vi "Convert to Waveforms (Multiple Lines).vi"(0 "data in":sgl[][](array[numeric]) format="%#.21g", 2 "reset? (F)":bool, 5 "sample rate [Hz]":sgl=9600.0 format="%#.6g", 7 "timestamp":timestamp, 9 "system info in":refnum<class "EP System Info.lvclass">, 11 "error in (no error)":errorcluster) -> (4 "voltage waveforms":waveform(dbl)[](array[waveform]), 6 "current waveforms":waveform(dbl)[](array[waveform]), 10 "system info out":refnum<class "EP System Info.lvclass">, 14 "interval length [s]":dbl, 15 "error out":errorcluster)   [LabVIEW 2014, in "NI_EP_Power Quality.lvlib"]
doc: "Converts resampled voltage and current data to voltage and current waveforms of different line configurations. This VI also arranges the order of the elements in the waveforms of each three-phase electrical power system for further measurement. For example, the orders are A-B-C-N for the four-channel method and A-B-C for the three-channel method. You must manually select the polymorphic instance you want to use."
uses:
  <vilib>/addons/Electrical Power/PQ/NI_EP_Power Quality.lvlib
  <vilib>/addons/Electrical Power/PQ/Common/Classes/System Info/EP System Info.lvclass
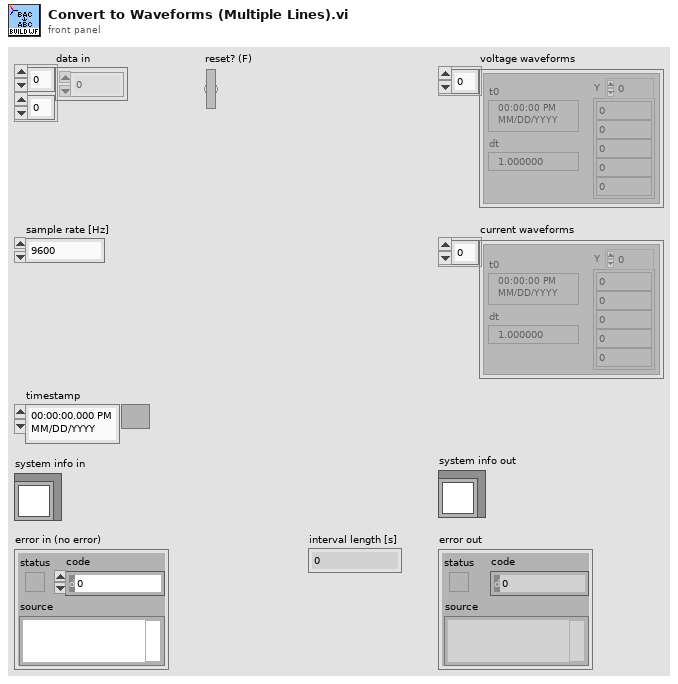
[diagram p1: front panel]
types:
  T1 = typedef "NI_EP_Power Quality.lvlib/ep_Channels Config.ctl" = cluster{"3-phase system ID":string, "physical channels":cluster{"channel phase":T2, "physical channel index":u16}[]}
  T2 = typedef "NI_EP_Power Quality.lvlib/ep_Channel Phase.ctl" = u16
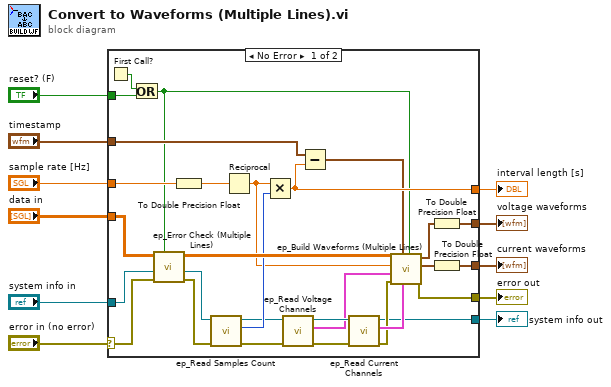
[diagram p0: block diagram]
diagram:
  n1 = case shown="No Error" "error in (no error)" {
    selector: "error in (no error)" -> [w32 w42]
    tunnel: "sample rate [Hz]" -> [w40 _]
    tunnel: "timestamp" -> [w39 _]
    tunnel: [w38 _] -> w9
    tunnel: [w24 _] -> w8
    tunnel: [w23 _] -> w7
    tunnel: "data in" -> [w31 _]
    tunnel: [w35 w42] -> w5
    tunnel: [w16 w41] -> w4
    tunnel: "reset? (F)" -> [w28 _]
    tunnel: "system info in" -> [w29 w41]
    frame No Error {
      n2 = First Call?() -> (First Call?: T/F=w33:bool)
      n3 = Or(x=w33, y=w28) -> (x .or. y?=w12:bool)
      n4 = call <vilib>:"ep_Error Check (Multiple Lines).vi"("reset? (F)"=w12, "error in (no error)"=w32, "system info in"=w29, "data in"=w31) -> ("error out"=w26:errorcluster, "system info out"=w27:refnum<class "EP System Info.lvclass">, "data out"=w30:sgl[][])  [unwired: 5 in]
      n5 = To Double Precision Float(number=w40) -> (double precision float=w34:dbl)
      n6 = call <vilib>:"ep_Read Samples Count.vi"("error in (no error)"=w26, "system info in"=w27) -> ("error out"=w20:errorcluster, "basic calc. interval (samples)"=w25:i32, "system info out"=w22:refnum<class "EP System Info.lvclass">)  [unwired: 5 in, 2 out]
      n7 = Reciprocal(x=w34) -> (1/x=w15:dbl)
      n8 = Multiply(x=w15, y=w25) -> (x*y=w38:dbl)
      n9 = call <vilib>:"ep_Read Voltage Channels.vi"("error in (no error)"=w20, "system info in"=w22) -> ("error out"=w19:errorcluster, "voltage channels"=w13:T1[], "system info out"=w21:refnum<class "EP System Info.lvclass">)  [unwired: 7 in]
      n10 = Subtract(x=w39, y=w38) -> (x-y=w14:timestamp)
      n11 = call <vilib>:"ep_Read Current Channels.vi"("error in (no error)"=w19, "system info in"=w21) -> ("error out"=w17:errorcluster, "current channels"=w18:T1[], "system info out"=w16:refnum<class "EP System Info.lvclass">)  [unwired: 7 in]
      n12 = call <vilib>:"ep_Build Waveforms (Multiple Lines).vi"("reset? (F)"=w12, "current channels"=w18, "t0"=w14, "error in (no error)"=w17, "voltage channels"=w13, "dt"=w15, "AI data"=w30) -> ("error out"=w35:errorcluster, "current waveforms"=w36:waveform(sgl)[], "voltage waveforms"=w37:waveform(sgl)[])  [unwired: 2 in]
      n13 = To Double Precision Float(number=w37) -> (double precision float=w24:waveform(dbl)[])
      n14 = To Double Precision Float(number=w36) -> (double precision float=w23:waveform(dbl)[])
    }
    frame Error {
    }
  }
  "voltage waveforms" <- w8
  "error out" <- w5
  "current waveforms" <- w7
  "system info out" <- w4
  "interval length [s]" <- w9
